vi "InsertItemArray.vi"(8 "Error":errorcluster, 9 "Mode":T2(ring), 10 "TreeItems[]":T1(array[cluster]), 11 "Tree in":refnum<class "Tree.lvclass">) -> (0 "Error":errorcluster, 3 "Tree out":refnum<class "Tree.lvclass">)   [LabVIEW 2021, in "Tree.lvlib" / "Tree.lvclass"]
uses:
  Tree.lvclass
  Private/TreeControllerTag.ctl
  Tree.lvclass/Tree.ctl
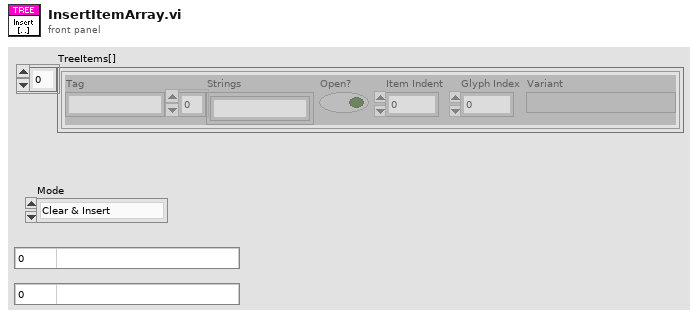
[diagram p1: front panel]
types:
  T1 = cluster{"Tag":string, "Strings":string[], "Open?":bool, "Item Indent":i32, "Glyph Index":i32, "Variant":variant}[]
  T2 = enum16{"Clear & Insert", "Update Existing", "Add to End"}
  T3 = typedef "Tree.lvlib/Tree.lvclass/TreeControllerTag.ctl" = enum8{"Null", "1. Add item", "2. Delete item", "3. Get All Tree Data", "4. Drag Starting", "5. Drag Ended", "6. Add Tree Values", "7. Get Item Value", "8. Edit Item", "9. StepBack", "10. Filter"}
  T4 = cluster{"TreeItems[]":cluster{"Tag":string, "Strings":string[], "Open?":bool, "Item Indent":i32, "Glyph Index":i32, "Variant":variant}[], "Mode":enum16{"Clear & Insert", "Update Existing", "Add to End"}}
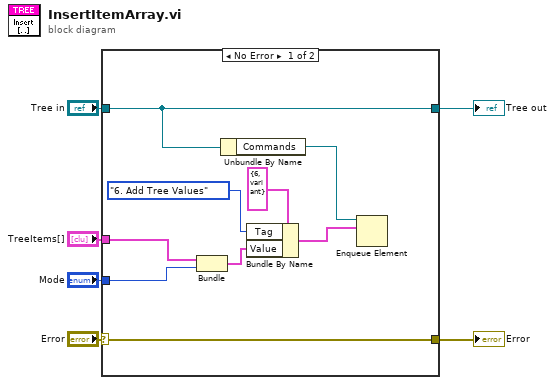
[diagram p0: block diagram]
diagram:
  n1 = case shown="No Error" "Error" {
    selector: "Error" -> [w15 w17]
    tunnel: [w15 w17] -> w5
    tunnel: [w14 w16] -> w3
    tunnel: "Tree in" -> [w14 w16]
    tunnel: "Mode" -> [w10 _]
    tunnel: "TreeItems[]" -> [w8 _]
    frame No Error {
      n2 = Bundle("TreeItems[]"=w8, "Mode"=w10) -> (w9:T4)  [unwired: 1 in]
      n3 = Unbundle By Name(w14) -> ("Commands"=w11:refnum<queue>)
      n4 = Bundle By Name(cluster=cluster{"Tag":u8, "Value":variant} {"Tag"=6, "Value"=variant} ("element"), "Tag"=TreeControllerTag."6. Add Tree Values", "Value"=w9) -> (w12:cluster{"Tag":u8, "Value":variant})
      n5 = Enqueue Element(queue=w11, element=w12) -> ()  [unwired: 2 in, 3 out]
    }
    frame Error {
    }
  }
  "Error" <- w5
  "Tree out" <- w3
